vi "Fetch Waveform.vi"(8 "error in (no error)":errorcluster, 9 "Timeout (10000 ms)":u32=10000, 10 "Channel (1: Channel 1)":u16(ring)=1 items=["Channel 1"=1, "Channel 2"=2], 11 "VISA resource name":refnum<visa-resource-name>) -> (0 "error out":errorcluster, 2 "Waveform Data":waveform(dbl)(graph), 3 "VISA resource name out":refnum<visa-resource-name>)   [LabVIEW 2015, in "Template - Scope.lvlib"]
doc: "Returns the waveform the oscilloscope acquired for the specified channel. The waveform is from an acquisition that you initiate prior to calling this VI.\n\nYou use the <b>Initiate</b> VI to start an acquisition on the channels that you enable with the <b>Configure Channel</b> VI. The oscilloscope acquires waveforms for the enabled channels concurrently. You must call this VI separately for each enabled channel to obtain the waveforms.\n\nYou can call the <b>Read Waveform</b> VI instead of using low-level VIs.\n\n<B>Note:</B> Use this VI only with other low-level VIs. The high-level VIs automatically incorporate this functionality. This VI does not check the instrument status."
uses:
  <instrlib>/_Template - Scope/Template - Scope.lvlib
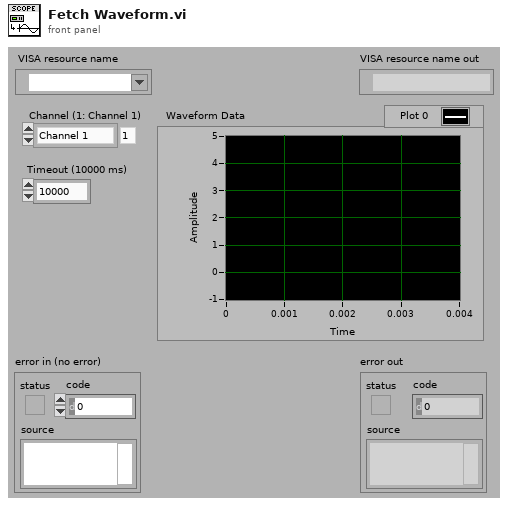
[diagram p1: front panel]
types:
  T1 = enum16{"big-endian, network order", "native, host order", "little-endian"}
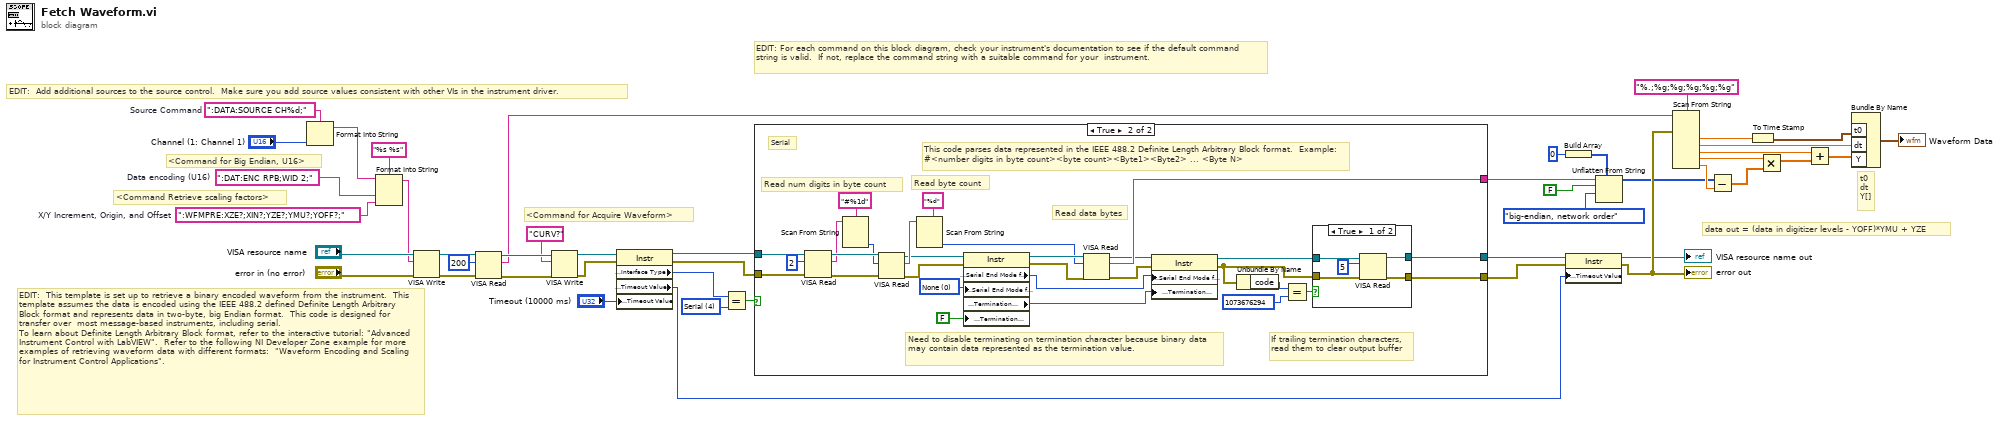
[diagram p0: block diagram]
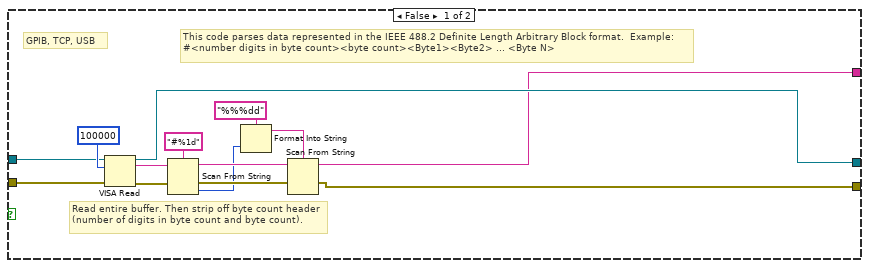
[diagram p2: hidden frame]
diagram:
  w2 = ":DAT:ENC RPB;WID 2;"  # Data encoding (U16)
  w23 = u16 4 items=["GPIB"=1, "VXI"=2, "GPIB-VXI"=3, "Serial"=4, "PXI"=5, "TCPIP"=6, "USB"=7] ("Interface Information:Interface Type")
  w31 = ":DATA:SOURCE CH%d;"  # Source Command
  w1 = ":WFMPRE:XZE?;XIN?;YZE?;YMU?;YOFF?;"  # X/Y Increment, Origin, and Offset
  # "<Command for Big Endian, U16>"
  # "data out = (data in digitizer levels - YOFF)*YMU + YZE"
  # "EDIT:  This template is set up to retrieve a binary encoded waveform from the instrument.  This template assumes the data is encoded using the IEEE 488.2 defined Definite Length Arbitrary Block format and represents data in two-byte, big Endian format.  This code is designed for transfer over  most message-based instruments, including serial. \nTo learn about Definite Length Arbitrary Block format, refer to the interactive tutorial: \"Advanced Instrument Control with LabVIEW\".  Refer to the following NI Developer Zone example for more examples of retrieving waveform data with different formats:  \"Waveform Encoding and Scaling for Instrument Control Applications\"."
  # "<Command for Acquire Waveform>"
  # "<Command Retrieve scaling factors>"
  # "t0\ndt\nY[]"
  # "EDIT:  Add additional sources to the source control.  Make sure you add source values consistent with other VIs in the instrument driver."
  # "EDIT: For each command on this block diagram, check your instrument's documentation to see if the default command string is valid.  If not, replace the command string with a suitable command for your  instrument."
  n1 = Format Into String(format string=w31, "Channel (1: Channel 1)") -> (resulting string=w28:string)  [unwired: 2 in, 1 out]
  n2 = Format Into String(format string="%s %s", initial string=w28, w2, w1) -> (resulting string=w27:string)  [unwired: 1 in, 1 out]
  n3 = VISA Write(VISA resource name="VISA resource name", write buffer=w27, error in (no error)="error in (no error)") -> (VISA resource name out=w46:refnum<visa-resource-name>, error out=w45:errorcluster)  [unwired: 1 out]
  n4 = VISA Read(VISA resource name=w46, byte count=u32 200, error in (no error)=w45) -> (VISA resource name out=w43:refnum<visa-resource-name>, read buffer=w36:string, error out=w42:errorcluster)  [unwired: 1 out]
  n5 = VISA Write(VISA resource name=w43, write buffer="CURV?", error in (no error)=w42) -> (VISA resource name out=w14:refnum<visa-resource-name>, error out=w22:errorcluster)  [unwired: 1 out]
  n6 = property class="Instr"(reference=w14, error in=w22, "General Settings:Timeout Value"="Timeout (10000 ms)") -> (reference out=w13:refnum<visa-resource-name>, error out=w21:errorcluster, "Interface Information:Interface Type"=w24:u16, "General Settings:Timeout Value"=w15:u32)
  n7 = Equal?(x=w24, y=w23) -> (x = y?=w20:bool)
  n8 = case shown="True" w20 {
    tunnel: w13 -> [w51 w89]
    tunnel: w21 -> [w50 w88]
    tunnel: [w48 w77] -> w18
    tunnel: [w49 w76] -> w19
    tunnel: [w47 w75] -> w6
    frame False {
      # "Read entire buffer. Then strip off byte count header (number of digits in byte count and byte count)."
      # "This code parses data represented in the IEEE 488.2 Definite Length Arbitrary Block format.  Example:  #<number digits in byte count><byte count><Byte1><Byte2> ... <Byte N>"
      # "GPIB, TCP, USB"
      n9 = VISA Read(VISA resource name=w51, byte count=u32 100000, error in (no error)=w50) -> (VISA resource name out=w49:refnum<visa-resource-name>, read buffer=w54:string, error out=w52:errorcluster)  [unwired: 1 out]
      n10 = Scan From String(format string="#%1d", input string=w54, error in=w52) -> (remaining string=w58:string, error out=w56:errorcluster, output 1=w55:i32)  [unwired: 2 in, 1 out]
      n11 = Format Into String(format string="%%%dd", w55) -> (resulting string=w57:string)  [unwired: 2 in, 1 out]
      n12 = Scan From String(format string=w57, input string=w58, error in=w56) -> (remaining string=w47:string, error out=w48:errorcluster)  [unwired: 3 in, 1 out]
    }
    frame True {
      w66 = u16 0 items=["None", "Last Bit", "TermChar"] ("Serial Settings:Serial End Mode for Reads")
      # "Read data bytes"
      # "Read num digits in byte count"
      # "Read byte count"
      # "This code parses data represented in the IEEE 488.2 Definite Length Arbitrary Block format.  Example:  #<number digits in byte count><byte count><Byte1><Byte2> ... <Byte N>"
      # "Need to disable terminating on termination character because binary data may contain data represented as the termination value."
      # "Serial"
      # "If trailing termination characters, read them to clear output buffer"
      n13 = VISA Read(VISA resource name=w89, byte count=u32 2, error in (no error)=w88) -> (VISA resource name out=w84:refnum<visa-resource-name>, read buffer=w74:string, error out=w85:errorcluster)  [unwired: 1 out]
      n14 = Scan From String(format string="#%1d", input string=w74) -> (output 1=w83:i32)  [unwired: 3 in, 3 out]
      n15 = VISA Read(VISA resource name=w84, byte count=w83, error in (no error)=w85) -> (VISA resource name out=w64:refnum<visa-resource-name>, read buffer=w82:string, error out=w63:errorcluster)  [unwired: 1 out]
      n16 = Scan From String(format string="%d", input string=w82) -> (output 1=w65:i32)  [unwired: 3 in, 3 out]
      n17 = property class="Instr"(reference=w64, error in=w63, "Serial Settings:Serial End Mode for Reads"=w66, "Message Based Settings:Termination Character Enable"=FALSE) -> (reference out=w70:refnum<visa-resource-name>, error out=w71:errorcluster, "Serial Settings:Serial End Mode for Reads"=w69:u16, "Message Based Settings:Termination Character Enable"=w62:bool)
      n18 = VISA Read(VISA resource name=w70, byte count=w65, error in (no error)=w71) -> (VISA resource name out=w68:refnum<visa-resource-name>, read buffer=w75:string, error out=w67:errorcluster)  [unwired: 1 out]
      n19 = property class="Instr"(reference=w68, error in=w67, "Serial Settings:Serial End Mode for Reads"=w69, "Message Based Settings:Termination Character Enable"=w62) -> (reference out=w73:refnum<visa-resource-name>, error out=w72:errorcluster)
      n20 = Unbundle By Name(w72) -> ("code"=w80:i32)
      n21 = Equal?(x=w80, y=1073676294 ("code")) -> (x = y?=w78:bool)
      n22 = case shown="True" w78 {
        tunnel: w73 -> [w94 w96]
        tunnel: w72 -> [w90 w95]
        tunnel: [w92 w96] -> w76
        tunnel: [w91 w95] -> w77
        frame True {
          n23 = VISA Read(VISA resource name=w94, byte count=u32 5, error in (no error)=w90) -> (VISA resource name out=w92:refnum<visa-resource-name>, error out=w91:errorcluster)  [unwired: 2 out]
        }
        frame False {
        }
      }
    }
  }
  n24 = Build Array(u16 0) -> (w3:u16[])
  n25 = property class="Instr"(reference=w19, error in=w18, "General Settings:Timeout Value"=w15) -> (reference out=→"VISA resource name out":refnum<visa-resource-name>, error out=w17:errorcluster)
  "error out" <- w17
  n26 = Unflatten From String(type=w3, binary string=w6, data includes array or string size? (T)=FALSE, byte order (0:big-endian, network order)=T1."big-endian, network order") -> (value=w4:u16[])  [unwired: 1 in, 2 out]
  n27 = Scan From String(format string="%.;%g;%g;%g;%g;%g", input string=w36, error in=w17) -> (output 1=w40:dbl, output 2=w38:dbl, output 3=w8:dbl, output 4=w11:dbl, output 5=w12:dbl)  [unwired: 6 in, 3 out]
  n28 = Subtract(x=w4, y=w12) -> (x-y=w37:dbl[])
  n29 = To Time Stamp(1:w40) -> (0:w39:timestamp)
  n30 = Multiply(x=w11, y=w37) -> (x*y=w9:dbl[])
  n31 = Add(x=w8, y=w9) -> (x+y=w10:dbl[])
  n32 = Bundle By Name("t0"=w39, "dt"=w38, "Y"=w10) -> (→"Waveform Data":waveform(dbl))  [unwired: 1 in]
